vi "Launcher.vi"   [LabVIEW 2020]
uses:
  Interactor/Interactor.lvclass
  C:/Program Files/National Instruments/LabVIEW 2026/vi.lib/MGI/Panel Manager/Panel Actor/Panel Actor/Panel Actor.lvclass
  <vilib>/MGI/Panel Manager/Panel/Window Position/Reference Position/Ref VI/Ref VI.lvclass
  C:/Program Files/National Instruments/LabVIEW 2026/vi.lib/MGI/Panel Manager/Panel/Window Position/Window Position.lvclass
  <vilib>/MGI/Panel Manager/Panel Actor/Panel Actor/Panel Actor.lvclass
  <vilib>/MGI/Panel Manager/Panel/Panel.lvlib
  <vilib>/MGI/Panel Manager/Panel/Window Position/Reference Position/Horizontal Alignment.ctl
  <vilib>/MGI/Panel Manager/Panel/Window Position/Reference Position/Reference Position.lvclass
  <vilib>/MGI/Panel Manager/Panel/Window Position/Reference Position/Vertical Alignment.ctl
  <vilib>/MGI/Panel Manager/Panel/Window Position/Reference Position/Alignment.ctl
  <vilib>/MGI/Panel Manager/Panel Actor/Panel Actor/Launch Root Panel Window.vi
  <vilib>/MGI/Panel Manager/Panel/Window Position/Reference Position/Ref VI/Ref VI.vi
panel:
  # "LAUNCHER"
types:
  T1 = typedef "Panel.lvlib/Reference Position.lvclass/Alignment.ctl" = cluster{"Horizontal":T2, "Vertical":T3}
  T2 = typedef "Panel.lvlib/Reference Position.lvclass/Horizontal Alignment.ctl" = enum16{"Left", "Center", "Right"}
  T3 = typedef "Panel.lvlib/Reference Position.lvclass/Vertical Alignment.ctl" = enum16{"Top", "Center", "Bottom"}
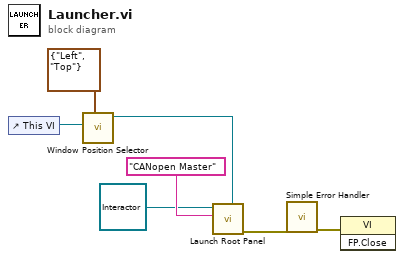
[diagram p0: block diagram]
diagram:
  n1 = control-ref of="This VI"() -> (w5:refnum<vi>)
  n2 = call-poly <vilib>:"Window Position Selector.vi"("Alignment"=T1 {"Horizontal"=enum."Left", "Vertical"=enum."Top"}, "Ref VI"=w5) -> ("Ref VI out"=w7:refnum<class "Ref VI.lvclass">)  [unwired: 8 in, 1 out]
  n3 = call-poly <vilib>:"Launch Root Panel.vi"("Window Position (Maximize First Call)"=w7, "Title"="CANopen Master", "Panel Actor in"=refnum<class "Interactor.lvclass"> refnum ("Interactor.lvlib:Interactor.lvclass")) -> ("Error Out"=w2:errorcluster)  [unwired: 7 in, 1 out]
  n4 = call <vilib>:"Simple Error Handler.vi"("error in (no error)"=w2) -> ("error out"=w1:errorcluster)  [unwired: 4 in, 4 out]
  n5 = invoke class="VI" method="FP.Close"(error in=w1) -> ()  [unwired: 2 in, 3 out]
